vi "VHM-continiousDataSet.vi"(8 "error in (no error)":errorcluster, 10 "Read Option":T1, 11 "VHM-VNA_Hardware_Manager in":refnum<class "VHM-VNA_Hardware_Manager.lvclass">) -> (0 "error out":errorcluster, 3 "VHM-VNA_Hardware_Manager out":refnum<class "VHM-VNA_Hardware_Manager.lvclass">)   [LabVIEW 2020, in "VHM-VNA_Hardware_Manager.lvlib" / "VHM-VNA_Hardware_Manager.lvclass"]
uses:
  VHM-VNA_Hardware_Manager.lvclass
  C:/Program Files (x86)/National Instruments/LabVIEW 2020/vi.lib/ActorFramework/Actor/Actor.lvclass
  VHM-continuous_get_clust.ctl
  VHM-VNA_Hardware_Manager.lvclass/VHM-VNA_Hardware_Manager.ctl
  VHM-VNA_Hardware_Manager Messages/VHM-getDataSet Msg/VHM-getDataSet Msg.lvclass
  C:/Program Files (x86)/National Instruments/LabVIEW 2020/vi.lib/ActorFramework/Message/Message.lvclass
  <vilib>/ActorFramework/Actor/Actor.lvclass/Actor.ctl
  <vilib>/ActorFramework/Message Enqueuer/Message Enqueuer.lvclass/Message Enqueuer.ctl
  <vilib>/ActorFramework/Message Enqueuer/Init from Existing Queue.vi
  <vilib>/ActorFramework/Message Enqueuer/Message Enqueuer.lvclass
  <vilib>/ActorFramework/Actor/Actor.lvclass
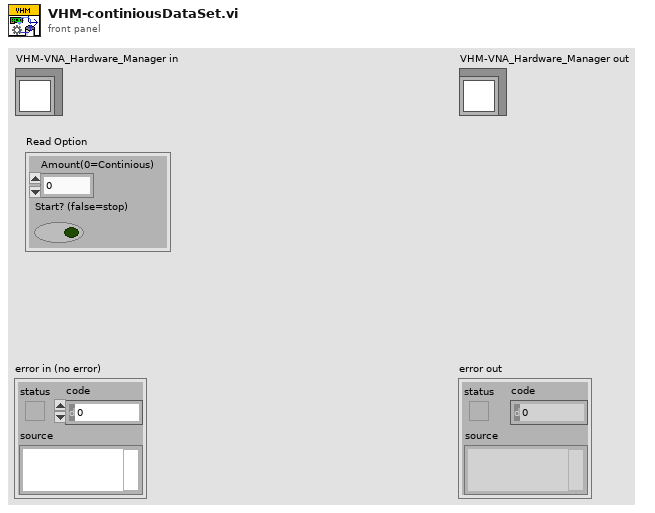
[diagram p1: front panel]
types:
  T1 = typedef "VHM-VNA_Hardware_Manager.lvlib/VHM-VNA_Hardware_Manager.lvclass/VHM-continuous_get_clust.ctl" = cluster{"Amount(0=Continious)":u8, "Start? (false=stop)":bool}
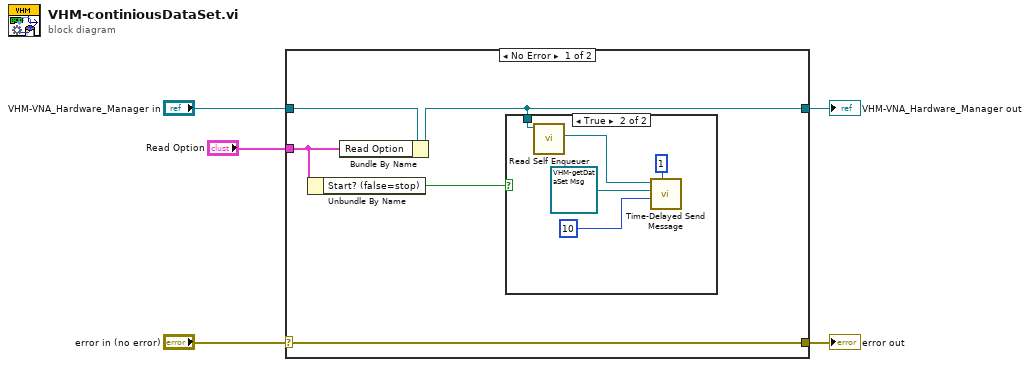
[diagram p0: block diagram]
diagram:
  n1 = case shown="No Error" "error in (no error)" {
    selector: "error in (no error)" -> [w9 w17]
    tunnel: [w9 w17] -> w4
    tunnel: [w7 w16] -> w2
    tunnel: "VHM-VNA_Hardware_Manager in" -> [w10 w16]
    tunnel: "Read Option" -> [w8 _]
    frame No Error {
      n2 = Unbundle By Name(w8) -> ("Start? (false=stop)"=w6:bool)
      n3 = Bundle By Name(cluster=w10, "Read Option"=w8) -> (w7:refnum<class "VHM-VNA_Hardware_Manager.lvclass">)
      n4 = case shown="True" w6 {
        tunnel: w7 -> [_ w15]
        frame False {
        }
        frame True {
          n5 = call <vilib>:"Read Self Enqueuer.vi"("Actor"=w15) -> ("Self Enqueuer"=w14:refnum<class "Message Enqueuer.lvclass">)  [unwired: 10 in]
          n6 = call <vilib>:"Time-Delayed Send Message.vi"("# Copies (0 = infinite repeat)"=u32 1, "Milliseconds To Wait"=10, "Message"=refnum<class "VHM-getDataSet Msg.lvclass"> refnum ("VHM-VNA_Hardware_Manager.lvlib:VHM-getDataSet Msg.lvclass"), "Message Enqueuer"=w14) -> ()  [unwired: 6 in, 2 out]
        }
      }
    }
    frame Error {
    }
  }
  "error out" <- w4
  "VHM-VNA_Hardware_Manager out" <- w2
